vi "Handle Messages.vi"(8 "error in (no error)":errorcluster, 9 "Message Data":variant, 10 "Message":string, 11 "Worker In":refnum<class "Worker.lvclass">) -> (0 "error out":errorcluster, 3 "Worker Out":refnum<class "Worker.lvclass">)   [LabVIEW 2020, in "Worker.lvclass"]
uses:
  Worker.lvclass
  C:/git/astemes-triarc-examples/source/Coffee Shop/Processes/People/Person/Person.lvclass
  C:/git/astemes-triarc-examples/source/Coffee Shop/Processes/People/Process Job/Job Handler.lvclass
  Process Job/Job Handler.lvclass
  Worker.lvclass/Worker.ctl
  Person/Person.lvclass
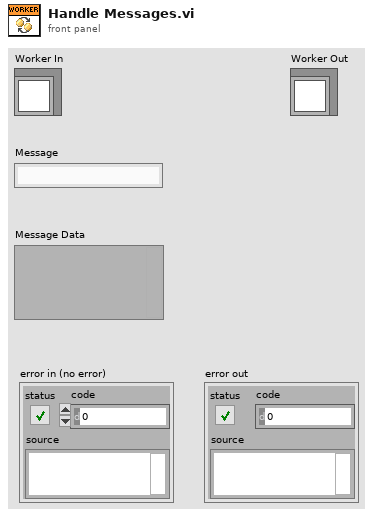
[diagram p1: front panel]
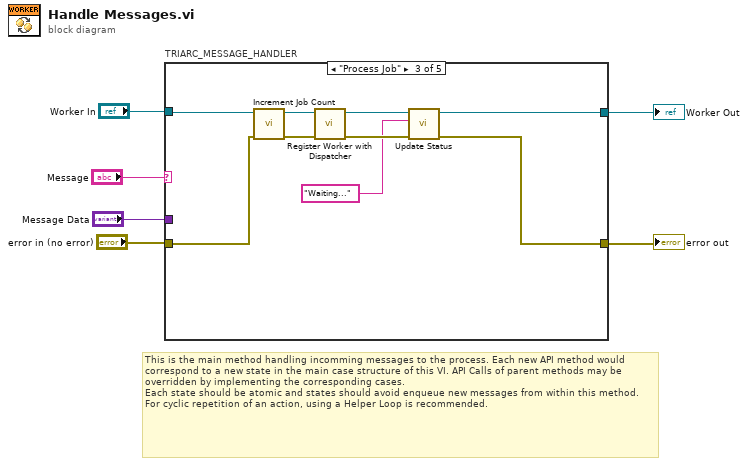
[diagram p0: block diagram]
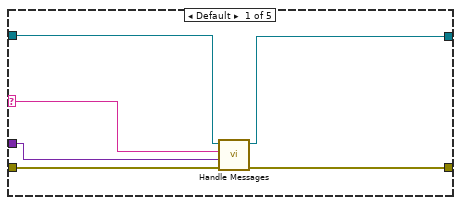
[diagram p2: hidden frame]
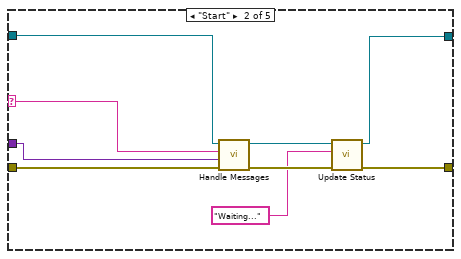
[diagram p3: hidden frame]
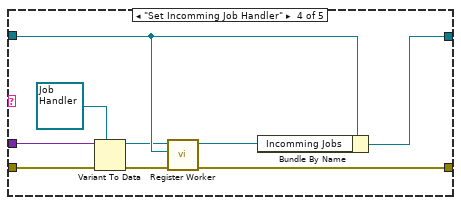
[diagram p4: hidden frame]
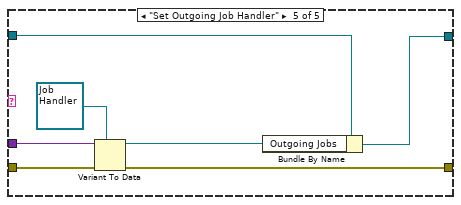
[diagram p5: hidden frame]
diagram:
  # "This is the main method handling incomming messages to the process. Each new API method would correspond to a new state in the main case structure of this VI. API Calls of parent methods may be overridden by implementing the corresponding cases.\nEach state should be atomic and states should avoid enqueue new messages from within this method. For cyclic repetition of an action, using a Helper Loop is recommended."
  n1 = case "TRIARC_MESSAGE_HANDLER" shown="\"Process Job\"" "Message" {
    selector: "Message" -> [w10 w19 _ _ _]
    tunnel: "error in (no error)" -> [w9 w18 w29 w39 w46]
    tunnel: "Worker In" -> [w12 w21 w30 w33 w41]
    tunnel: "Message Data" -> [w11 w20 _ w37 w44]
    tunnel: [w8 w16 w25 w35 w43] -> w2
    tunnel: [w7 w14 w23 w34 w42] -> w1
    frame Default {
      n2 = call-parent "Handle Messages.vi"("error in (no error)"=w9, "Message Data"=w11, "Message"=w10, "Person In"=w12) -> ("error out"=w8:errorcluster, "Person Out"=w7:refnum<class "Worker.lvclass">)  [unwired: 6 in]
    }
    frame "Start" {
      n3 = call-parent "Handle Messages.vi"("error in (no error)"=w18, "Message Data"=w20, "Message"=w19, "Person In"=w21) -> ("error out"=w17:errorcluster, "Person Out"=w15:refnum<class "Worker.lvclass">)  [unwired: 6 in]
      n4 = call "Update Status.vi"("error in (no error)"=w17, "Status"="Waiting...", "Person In"=w15) -> ("error out"=w16:errorcluster, "Person Out"=w14:refnum<class "Worker.lvclass">)  [unwired: 7 in]
    }
    frame "Process Job" {
      n5 = call "Increment Job Count.vi"("error in (no error)"=w29, "Worker In"=w30) -> ("error out"=w27:errorcluster, "Worker Out"=w28:refnum<class "Worker.lvclass">)  [unwired: 8 in]
      n6 = call "Register Worker with Dispatcher.vi"("error in (no error)"=w27, "Worker In"=w28) -> ("error out"=w26:errorcluster, "Worker Out"=w24:refnum<class "Worker.lvclass">)  [unwired: 8 in]
      n7 = call "Update Status.vi"("error in (no error)"=w26, "Status"="Waiting..." ("Message"), "Person In"=w24) -> ("error out"=w25:errorcluster, "Person Out"=w23:refnum<class "Worker.lvclass">)  [unwired: 7 in]
    }
    frame "Set Incomming Job Handler" {
      n8 = Variant To Data(error in=w39, type=refnum<class "Job Handler.lvclass"> refnum ("Process Job.lvclass"), Variant=w37) -> (data=w32:refnum<class "Job Handler.lvclass">, error out=w36:errorcluster)
      n9 = call-dynamic "Register Worker.vi"("error in (no error)"=w36, "Worker"=w33, "Job Handler In"=w32) -> ("error out"=w35:errorcluster, "Job Handler Out"=w31:refnum<class "Job Handler.lvclass">)  [unwired: 7 in]
      n10 = Bundle By Name(cluster=w33, "Incomming Jobs"=w31) -> (w34:refnum<class "Worker.lvclass">)
    }
    frame "Set Outgoing Job Handler" {
      n11 = Variant To Data(error in=w46, type=refnum<class "Job Handler.lvclass"> refnum ("Process Job.lvclass"), Variant=w44) -> (data=w40:refnum<class "Job Handler.lvclass">, error out=w43:errorcluster)
      n12 = Bundle By Name(cluster=w41, "Outgoing Jobs"=w40) -> (w42:refnum<class "Worker.lvclass">)
    }
  }
  "error out" <- w2
  "Worker Out" <- w1
